vi "Serialize.vi"(8 "error in":errorcluster, 9 "OwningElement in":refnum<k20>, 10 "Document in":refnum<k20>, 11 "CustomElement in":refnum<class "CustomElement.lvclass">) -> (0 "error out":errorcluster, 1 "OwningElement out":refnum<k20>, 2 "Document out":refnum<k20>, 3 "CustomElement out":refnum<class "CustomElement.lvclass">)   [LabVIEW 2021, in "ProligentXMLGenerator.lvlib" / "CustomElement.lvclass"]
uses:
  CustomElement.lvclass
  CustomElement.lvclass/CustomElement.ctl
  <resource>/objmgr/DOMUserDefRef.rc
  <vilib>/xml/NI_XML.lvlib
  <vilib>/xml/Close Reference(Node).vi
  Base/DOMSupport/DOMSupport.lvlib
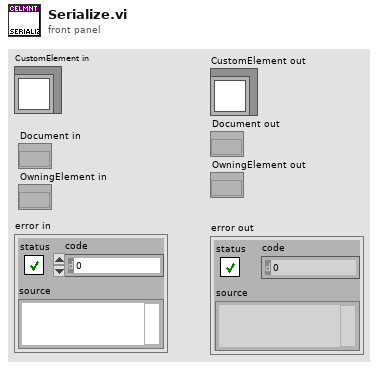
[diagram p1: front panel]
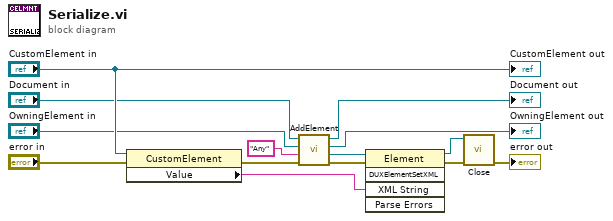
[diagram p0: block diagram]
diagram:
  n1 = property on="Property Node" class="CustomElement"(reference="CustomElement in", error in="error in") -> (error out=w5:errorcluster, "Value"=w1:string)  [unwired: 1 out]
  n2 = call "AddElement.vi"("error in"=w5, "Name"="Any" ("Tag Name"), "OwningElement in"="OwningElement in", "Document in"="Document in") -> ("error out"=w3:errorcluster, "NewElement"=w4:refnum<k20>, "OwningElement out"=→"OwningElement out":refnum<k20>, "Document out"=→"Document out":refnum<k20>)  [unwired: 4 in]
  n3 = invoke on="Invoke Node" class="Element" method="DUXElementSetXML"(reference=w4, error in=w3, "XML String"=w1) -> (reference out=w11:refnum<k20>, error out=w12:errorcluster)  [unwired: 2 in, 3 out]
  n4 = call-poly <vilib>:"Close.vi"("error in (no error)"=w12, "node"=w11) -> ("error out"=→"error out":errorcluster)  [unwired: 7 in]
  "CustomElement out" <- "CustomElement in"
